vi "GObjects Move.vi"(8 "error in (no error)":errorcluster, 10 "Relative Moves in":cluster{"Left":i32, "Top":i32}[](array[cluster]), 11 "GObjects in":refnum<vi>[](array[refnum])) -> (0 "error out":errorcluster, 3 "GObjects out":refnum<vi>[](array[refnum]))   [LabVIEW 2019, in "Builtins.lvlib"]
doc: "Moves the GObjects relative to current position.\n\nCreated by: Ryan Pacini"
uses:
  Builtins.lvlib
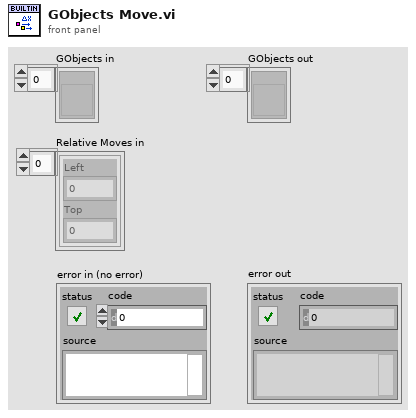
[diagram p1: front panel]
types:
  T1 = typedef "LVPositionTypeDef.ctl" = cluster{"Left":i32, "Top":i32}
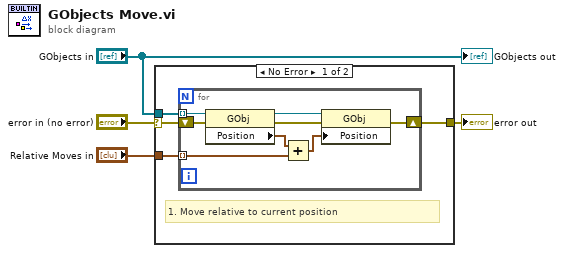
[diagram p0: block diagram]
diagram:
  n1 = case shown="No Error" "error in (no error)" {
    selector: "error in (no error)" -> [w7 w17]
    tunnel: [w8 w17] -> w3
    tunnel: "GObjects in" -> [w6 _]
    tunnel: "Relative Moves in" -> [w5 _]
    frame No Error {
      # "1. Move relative to current position"
      n2 = for {
        tunnel: w6 -> [w16] mode=indexing
        shift-right: [w15] -> w8
        shift-left: w7 -> [w13]
        tunnel: w5 -> [w9] mode=indexing
        n3 = property class="GObj"(reference=w16, error in=w13) -> (reference out=w14:refnum<vi>, error out=w12:errorcluster, "Position"=w11:T1)
        n4 = Add(x=w11, y=w9) -> (x+y=w10:T1)
        n5 = property class="GObj"(reference=w14, error in=w12, "Position"=w10) -> (error out=w15:errorcluster)  [unwired: 1 out]
      }
    }
    frame Error {
    }
  }
  "error out" <- w3
  "GObjects out" <- "GObjects in"
